vi "Stop.vi"(4 "Time":dbl=1.0, 6 "Stop Arm?":bool=TRUE, 11 "error in":errorcluster) -> (0 "Done":bool, 3 "error out":errorcluster)   [LabVIEW 2015]
uses:
  References/Refnums.vi
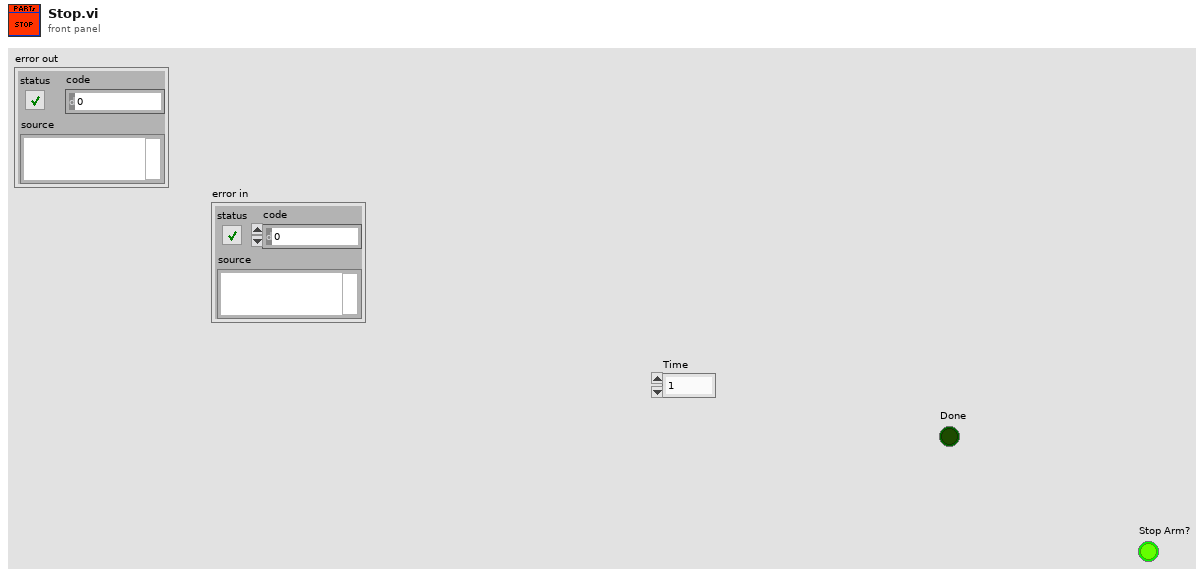
[diagram p1: front panel]
types:
  T1 = typedef "WPI_MotorControlDeviceRef.ctl" = cluster{"DeviceStatus":errorcluster, "Type":T2, "PWM":cluster{"PWM Channel":T3, "DeadBand":T4}, "CAN":cluster{"Device Number":u8, "Control Mode":T5, "Semaphore":T6, "Max Vout":dbl, "TalonSRX Control Mode":T7}, "Invert":bool}
  T2 = typedef "WPI_MotorControlType.ctl" = enum16{"PWM", "CAN", "CANTalonSRX"}
  T3 = typedef "FPGA_DIOPWMChannel.ctl" = enum8{"PWM 0", "PWM 1", "PWM 2", "PWM 3", "PWM 4", "PWM 5", "PWM 6", "PWM 7", "PWM 8", "PWM 9", "PWM MXP 0", "PWM MXP 1", "PWM MXP 2", "PWM MXP 3", "PWM MXP 4", "PWM MXP 5", "PWM MXP 6", "PWM MXP 7", "PWM MXP 8", "PWM MXP 9", "Invalid"}
  T4 = typedef "WPI_PWMDeadband.ctl" = cluster{"Name":string, "maxPositivePwm":i32, "minPositivePwm":i32, "centerPwm":i32, "maxNegativePwm":i32, "minNegativePwm":i32, "angularRange":u16}
  T5 = typedef "WPI_CANJaguar_ControlMode.ctl" = enum8{"Percent VBus", "Current", "Speed", "Position", "Voltage"}
  T6 = typedef "Semaphore RefNum" = refnum<k1>
  T7 = typedef "WPI_CANTalonSRX_APIControlMode.ctl" = enum8{"Percent VBus", "Speed", "Position", "Slave", "Unchanged / Invalid", "Voltage Compensation", "Current", "Motion Profile"}
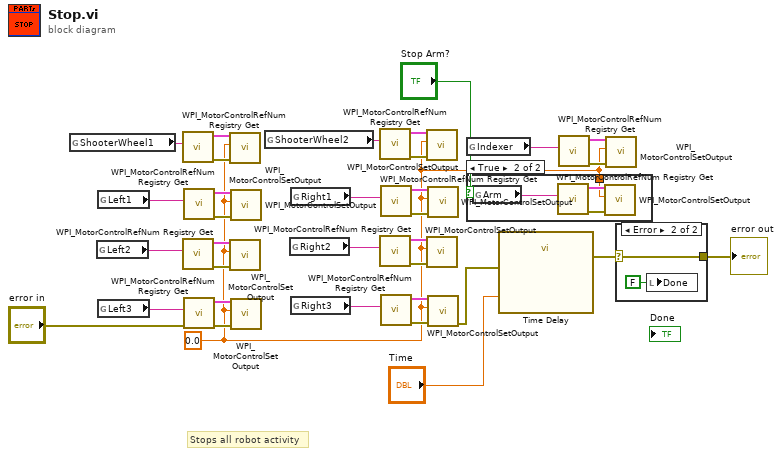
[diagram p0: block diagram]
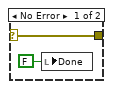
[diagram p3: hidden frame]
diagram:
  w2 = 0.0 ("Output")
  # "Stops all robot activity"
  n1 = global read "Refnums.vi" "ShooterWheel1"() -> (w11:string)
  n2 = global read "Refnums.vi" "Left2"() -> (w18:string)
  n3 = global read "Refnums.vi" "Left1"() -> (w17:string)
  n4 = global read "Refnums.vi" "Left3"() -> (w23:string)
  n5 = call <vilib>:"WPI_MotorControlRefNum Registry Get.vi"("refnum name"=w11) -> ("error out"=w13:errorcluster, "MotorControlDevRef"=w12:T1)  [unwired: 9 in]
  n6 = call <vilib>:"WPI_MotorControlRefNum Registry Get.vi"("refnum name"=w18) -> ("error out"=w20:errorcluster, "MotorControlDevRef"=w19:T1)  [unwired: 9 in]
  n7 = call <vilib>:"WPI_MotorControlRefNum Registry Get.vi"("refnum name"=w17) -> ("error out"=w15:errorcluster, "MotorControlDevRef"=w16:T1)  [unwired: 9 in]
  n8 = call <vilib>:"WPI_MotorControlRefNum Registry Get.vi"("error in (no error)"="error in", "refnum name"=w23) -> ("error out"=w21:errorcluster, "MotorControlDevRef"=w22:T1)  [unwired: 8 in]
  n9 = call <vilib>:"WPI_MotorControlSetOutput.vi"("error in (no error)"=w13, "Output"=w2, "MotorControlDevRef"=w12) -> ()  [unwired: 6 in, 3 out]
  n10 = call <vilib>:"WPI_MotorControlSetOutput.vi"("error in (no error)"=w20, "Output"=w2, "MotorControlDevRef"=w19) -> ()  [unwired: 6 in, 3 out]
  n11 = call <vilib>:"WPI_MotorControlSetOutput.vi"("error in (no error)"=w15, "Output"=w2, "MotorControlDevRef"=w16) -> ()  [unwired: 6 in, 3 out]
  n12 = call <vilib>:"WPI_MotorControlSetOutput.vi"("error in (no error)"=w21, "Output"=w2, "MotorControlDevRef"=w22) -> ()  [unwired: 6 in, 3 out]
  n13 = global read "Refnums.vi" "ShooterWheel2"() -> (w10:string)
  n14 = global read "Refnums.vi" "Right2"() -> (w29:string)
  n15 = global read "Refnums.vi" "Right1"() -> (w30:string)
  n16 = global read "Refnums.vi" "Right3"() -> (w24:string)
  n17 = call <vilib>:"WPI_MotorControlRefNum Registry Get.vi"("refnum name"=w10) -> ("error out"=w8:errorcluster, "MotorControlDevRef"=w9:T1)  [unwired: 9 in]
  n18 = call <vilib>:"WPI_MotorControlRefNum Registry Get.vi"("refnum name"=w29) -> ("error out"=w27:errorcluster, "MotorControlDevRef"=w28:T1)  [unwired: 9 in]
  n19 = call <vilib>:"WPI_MotorControlRefNum Registry Get.vi"("refnum name"=w30) -> ("error out"=w32:errorcluster, "MotorControlDevRef"=w31:T1)  [unwired: 9 in]
  n20 = call <vilib>:"WPI_MotorControlRefNum Registry Get.vi"("refnum name"=w24) -> ("error out"=w26:errorcluster, "MotorControlDevRef"=w25:T1)  [unwired: 9 in]
  n21 = call <vilib>:"WPI_MotorControlSetOutput.vi"("error in (no error)"=w8, "Output"=w2, "MotorControlDevRef"=w9) -> ()  [unwired: 6 in, 3 out]
  n22 = call <vilib>:"WPI_MotorControlSetOutput.vi"("error in (no error)"=w27, "Output"=w2, "MotorControlDevRef"=w28) -> ()  [unwired: 6 in, 3 out]
  n23 = call <vilib>:"WPI_MotorControlSetOutput.vi"("error in (no error)"=w32, "Output"=w2, "MotorControlDevRef"=w31) -> ()  [unwired: 6 in, 3 out]
  n24 = call <vilib>:"WPI_MotorControlSetOutput.vi"("error in (no error)"=w26, "Output"=w2, "MotorControlDevRef"=w25) -> ("error out"=w14:errorcluster)  [unwired: 6 in, 2 out]
  n25 = global read "Refnums.vi" "Indexer"() -> (w7:string)
  n26 = case shown="True" "Stop Arm?" {
    tunnel: w2 -> [_ w35]
    frame False {
    }
    frame True {
      n27 = global read "Refnums.vi" "Arm"() -> (w36:string)
      n28 = call <vilib>:"WPI_MotorControlRefNum Registry Get.vi"("refnum name"=w36) -> ("error out"=w38:errorcluster, "MotorControlDevRef"=w37:T1)  [unwired: 9 in]
      n29 = call <vilib>:"WPI_MotorControlSetOutput.vi"("error in (no error)"=w38, "Output"=w35, "MotorControlDevRef"=w37) -> ()  [unwired: 6 in, 3 out]
    }
  }
  n30 = call "Time Delay"("error in (no error)"=w14, "Delay Time (s)"="Time") -> ("error out"=w4:errorcluster)  [unwired: 9 in]
  n31 = call <vilib>:"WPI_MotorControlRefNum Registry Get.vi"("refnum name"=w7) -> ("error out"=w5:errorcluster, "MotorControlDevRef"=w6:T1)  [unwired: 9 in]
  n32 = call <vilib>:"WPI_MotorControlSetOutput.vi"("error in (no error)"=w5, "Output"=w2, "MotorControlDevRef"=w6) -> ()  [unwired: 6 in, 3 out]
  n33 = case shown="Error" w4 {
    selector: w4 -> [w40 w42]
    tunnel: [w40 w42] -> w3
    frame No Error {
      n34 = local write "Done"(FALSE ("Done")) -> ()
    }
    frame Error {
      n35 = local write "Done"(FALSE ("Done")) -> ()
    }
  }
  "error out" <- w3
